vi "Close Facade.vi"(8 "error in":errorcluster, 11 "cPAS Facade in":refnum<class "cPAS Facade.lvclass">) -> (0 "error out":errorcluster, 3 "cPAS Facade out":refnum<class "cPAS Facade.lvclass">)   [LabVIEW 2015, in "cPAS Facade.lvclass"]
doc: "Send the stop signal to the open UIs, close the data references, remove the current VI from the subpanel and close the reference to all of the panels."
uses:
  cPAS Facade.lvclass
  Reusable/GUI/Facade/GUI Facade.lvclass
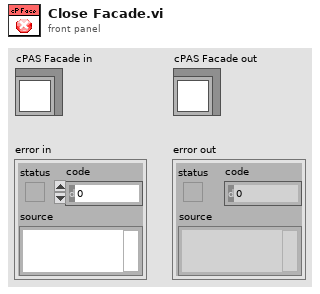
[diagram p1: front panel]
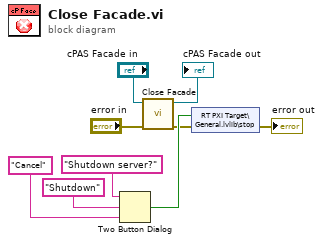
[diagram p0: block diagram]
diagram:
  n1 = Two Button Dialog(message="Shutdown server?", 1:"Cancel" ("F button name (\"Cancel\")"), 2:"Shutdown" ("T button name (\"OK\")")) -> (T button?=w4:bool)
  n2 = call-parent "Close Facade.vi"("error in"="error in", "GUI Facade in"="cPAS Facade in") -> ("error out"=w3:errorcluster, "GUI Facade out"=→"cPAS Facade out":refnum<class "cPAS Facade.lvclass">)  [unwired: 8 in]
  n3 = shared-variable "RT PXI Target\\General.lvlib\\stop"(w4, error in=w3) -> (error out=→"error out":errorcluster)
